vi "getNineAddrInMemroy(n+1).vi"(0 "col":u16, 5 "row":u16, 7 "Width":u16, 11 "divider":u8) -> (1 "1":u16, 2 "2":u16, 3 "3":u16, 4 "4":u16, 8 "5":u16, 12 "7":u16, 13 "8":u16, 14 "9":u16, 15 "6":u16)   [LabVIEW 2016]
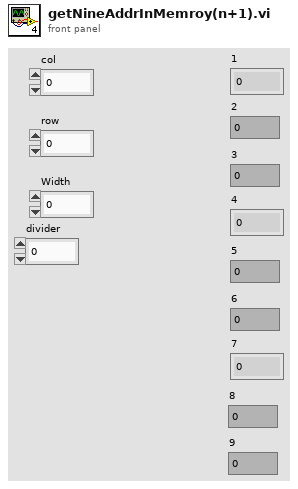
[diagram p1: front panel]
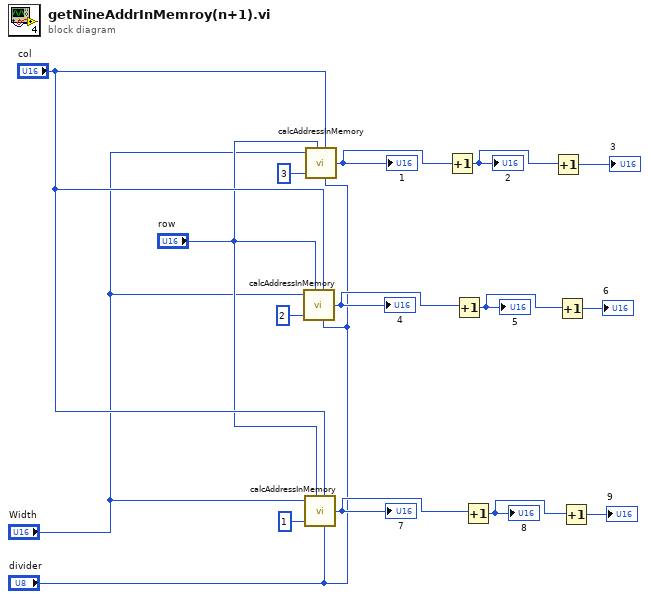
[diagram p0: block diagram]
diagram:
  n1 = call "calcAddressInMemory.vi"("Width"="Width", "Rows"="row", "delayRowCount"=u16 2, "Cols"="col", "divider"="divider") -> ("addressInMemory"=w10:u16)  [unwired: 4 in]
  "4" <- w10
  n2 = call "calcAddressInMemory.vi"("Width"="Width", "Rows"="row", "delayRowCount"=u16 1, "Cols"="col", "divider"="divider") -> ("addressInMemory"=w6:u16)  [unwired: 4 in]
  "7" <- w6
  n3 = call "calcAddressInMemory.vi"("Width"="Width", "Rows"="row", "delayRowCount"=u16 3, "Cols"="col", "divider"="divider") -> ("addressInMemory"=w13:u16)  [unwired: 4 in]
  "1" <- w13
  n4 = Increment(x=w13) -> (x+1=w14:u16)
  "2" <- w14
  n5 = Increment(x=w10) -> (x+1=w11:u16)
  "5" <- w11
  n6 = Increment(x=w6) -> (x+1=w7:u16)
  "8" <- w7
  n7 = Increment(x=w14) -> (x+1=→"3":u16)
  n8 = Increment(x=w11) -> (x+1=→"6":u16)
  n9 = Increment(x=w7) -> (x+1=→"9":u16)
